vi "waveform-to-XY (SubVI).vi"(2 "waveform":waveform(dbl), 3 "offset of cut":dbl, 4 "cut x-axis format":u16) -> (0 "Y":dbl[](array[numeric]), 1 "X":dbl[](array[numeric]))   [LabVIEW 2014]
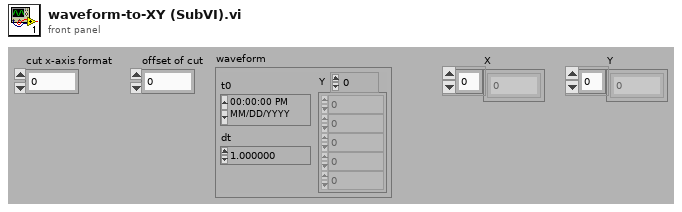
[diagram p1: front panel]
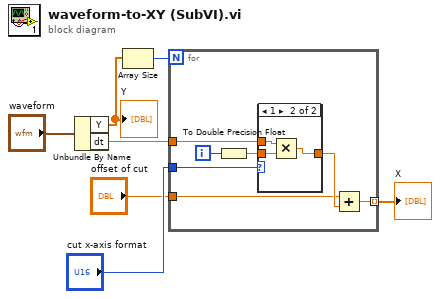
[diagram p0: block diagram]
diagram:
  n1 = Unbundle By Name("waveform") -> ("Y"=w1:dbl[], "dt"=w6:dbl)
  "Y" <- w1
  n2 = Array Size(array=w1) -> (size(s)=w3:i32)
  n3 = for {
    N: w3 -> [_]
    tunnel: w6 -> [w14]
    tunnel: "offset of cut" -> [w12]
    tunnel: [w11] -> w2 mode=indexing
    tunnel: "cut x-axis format" -> [w8]
    i -> [w9]
    n4 = To Double Precision Float(number=w9) -> (double precision float=w10:dbl)
    n5 = case shown="1" w8 {
      tunnel: w14 -> [_ w18]
      tunnel: [w15 w17] -> w13
      tunnel: w10 -> [w15 w16]
      frame 0, Default {
      }
      frame 1 {
        n6 = Multiply(x=w18, y=w16) -> (x*y=w17:dbl)
      }
    }
    n7 = Add(x=w12, y=w13) -> (x+y=w11:dbl)
  }
  "X" <- w2
